vi "DVS_LabVIEW_Controller - Copy.vi"() -> ()   [LabVIEW 2013]
doc: "This example demonstrates temperature control and monitoring.\n\nNote:\nBefore start this VI is it necessary:\n\n- preconfigure some specific parameters that are not supported by this driver (e.g. PV-I/O Type, Linearization type, Alarm Input Values... ) by Quick Codes, or by Eurotherm iTools or by instrument front panel controls\n- enter correct VISA Resource Descriptor, Device Address and Baud Rate into front-panel controls"
uses:
  <vilib>/Instr/_visa.llb/VISA Event Mechanism.ctl
  <vilib>/Instr/_visa.llb/Select Event Type.ctl
  <vilib>/DAQmx/read.llb/DAQmx Read (Analog DBL 1Chan 1Samp).vi
  <vilib>/Utility/file.llb/Write To Spreadsheet File (string).vi
  <vilib>/Instr/_visa.llb/VISA Configure Serial Port (Instr).vi
  <vilib>/DAQmx/miscellaneous.llb/DAQmx Fill In Error Info.vi
  <instrlib>/Keithley 24XX/Public/Data/Read (Single Point).vi
  <instrlib>/Keithley 24XX/Keithley 24XX.lvlib
panel:
  in  "stop":bool
  in  "Tab Control":T1(tab)
  in  "Add comments to the data file here and click anywhere outside\nthe comment box to save. The time at which the comment is\nsaved is recorded in the data file.":string
  in  "O2 PUMP":bool
  in  "QCM":bool
  out "Program Errors":errorcluster
  out "Starting Date/Time":string
  in  "Keithley 4200":bool
  in  "Keithley 2420":bool
  in  "J-KEM":bool
  in  "Automatically stop\nmeasurement?":bool
  in  "Stop after elapsed minutes":dbl
  out "Time Elapsed (min)":dbl caption="Elapsed Time (s)"
  in  "RapidOX":bool
  out "Freq and Resistance Graph 2":T2(graph)
  out "Frequency (Hz)":dbl format="%.6e"
  out "Resistance (Ohm)":dbl format="%.6e"
  out "Waveform Chart 5":cluster{dbl, dbl}(graph)
  out "Current Temp (C)":dbl
  in  "Temp Setpoint (C)":dbl=25.0
  out "Current Setpoint (C)":dbl
  out "Waveform Chart 2":dbl(graph)
  out "Waveform Chart":cluster{dbl}(graph)
  out "Torr":dbl
  out "%":dbl
  out "atm":dbl
  out "O2 pump voltage":dbl format="%0.2f"
  in  "Com Port":i32(ring) items=["Com 1", "Com 2", "Com 3", "Com 4", "Com 5", "Com 6", "COM 7", "COM 8", "COM 9", "COM 10", "COM 11", "COM 12", "com 13", "COM 14"]
  in  "Baud Rate 2":i32(ring)=2 items=["2400", "4800", "9600", "19200", "38400", "57600", "115200"]
  in  "Com Port 2":i32(ring) items=["Com 1", "Com 2", "Com 3", "Com 4", "Com 5", "Com 6", "COM 7", "COM 8", "COM 9", "COM 10", "COM 11", "COM 12", "com 13", "COM 14"]
  out "Waveform Chart 6":cluster{dbl}(graph)
  out "O2 Concentration (%)":dbl
  out "Waveform Chart 4":cluster{"Resistance":sgl}(graph)
  out "Resistance (Ohm)":sgl
  in  "Measurement":enum16{"Resistor/Diode", "Transistor"}(ring)
  out "Waveform Chart 3":cluster{dbl}(graph)
  out "XY Graph":cluster{dbl[], dbl[]}(graph)
  out "Current (A)    Voltage (V)":dbl[][](array[numeric]) caption="appended array"
  out "Resistance (Ohm)":dbl
  # "Configuring Instrument\n \nPlease Wait......\n\nChart will update in 20 sec"
  # "Instruments Connected"
  # "COMMENT BOX"
  # "Instructions:\nSelect the instruments above which are connected, turned on, and configured to record data.\nRun the Pirani Control software, and make sure Pirani is saving a log of the temp/pressure/gas flow data. \nClick the RUN arrow on the LabVIEW toolbar, and wait for instruments to begin recording.\nTo end, click the red STOP button ONLY for instruments that are running.\nDO NOT press the STOP button on the toolbar."
  # "O2 Partial\nPressure"
  # "V"
  # "4-Point Resistance Measurement:\nSMU1 = Current Source, Voltmeter\nSMU2 = COM & GND"
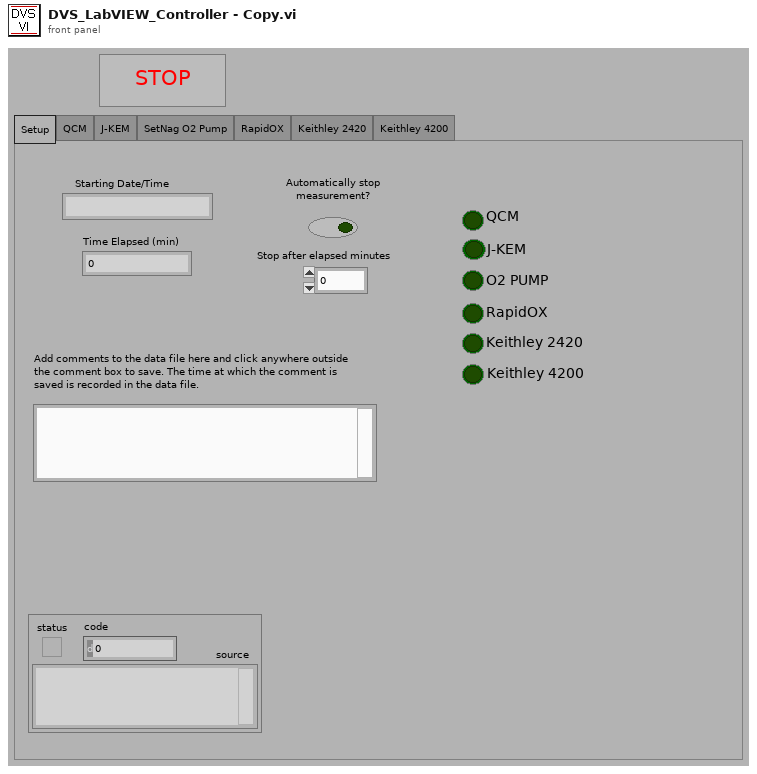
[diagram p1: front panel]
types:
  T1 = enum32{"Setup", "QCM", "J-KEM", "SetNag O2 Pump", "RapidOX", "Keithley 2420", "Keithley 4200"}
  T2 = cluster{"XY chart data":cluster{"x":dbl, "y":dbl}[]}[]
  T3 = enum16{"open", "open or create", "create or replace", "create", "open (read only)"}
  T4 = enum16{"no parity", "odd parity", "even parity", "mark parity", "space parity"}
  T5 = typedef "Select Event Type.ctl" = u32
  T6 = typedef "VISA Event Mechanism.ctl" = u16
  T7 = cluster{bool, "VISA resource name":refnum<visa-resource-name>, "error out":errorcluster}
  T8 = cluster{bool, "VISA resource name out":refnum<visa-resource-name>, "error out":errorcluster}
  T9 = cluster{"task out":refnum<k21>, "error out":errorcluster, bool}
  T10 = cluster{bool, "VISA out":refnum<visa-resource-name>, "error out":errorcluster}
  T11 = cluster{"timestamp out":dbl, "Frequency out":dbl}
  T12 = cluster{"timestamp out":dbl, "Resistance out":dbl}
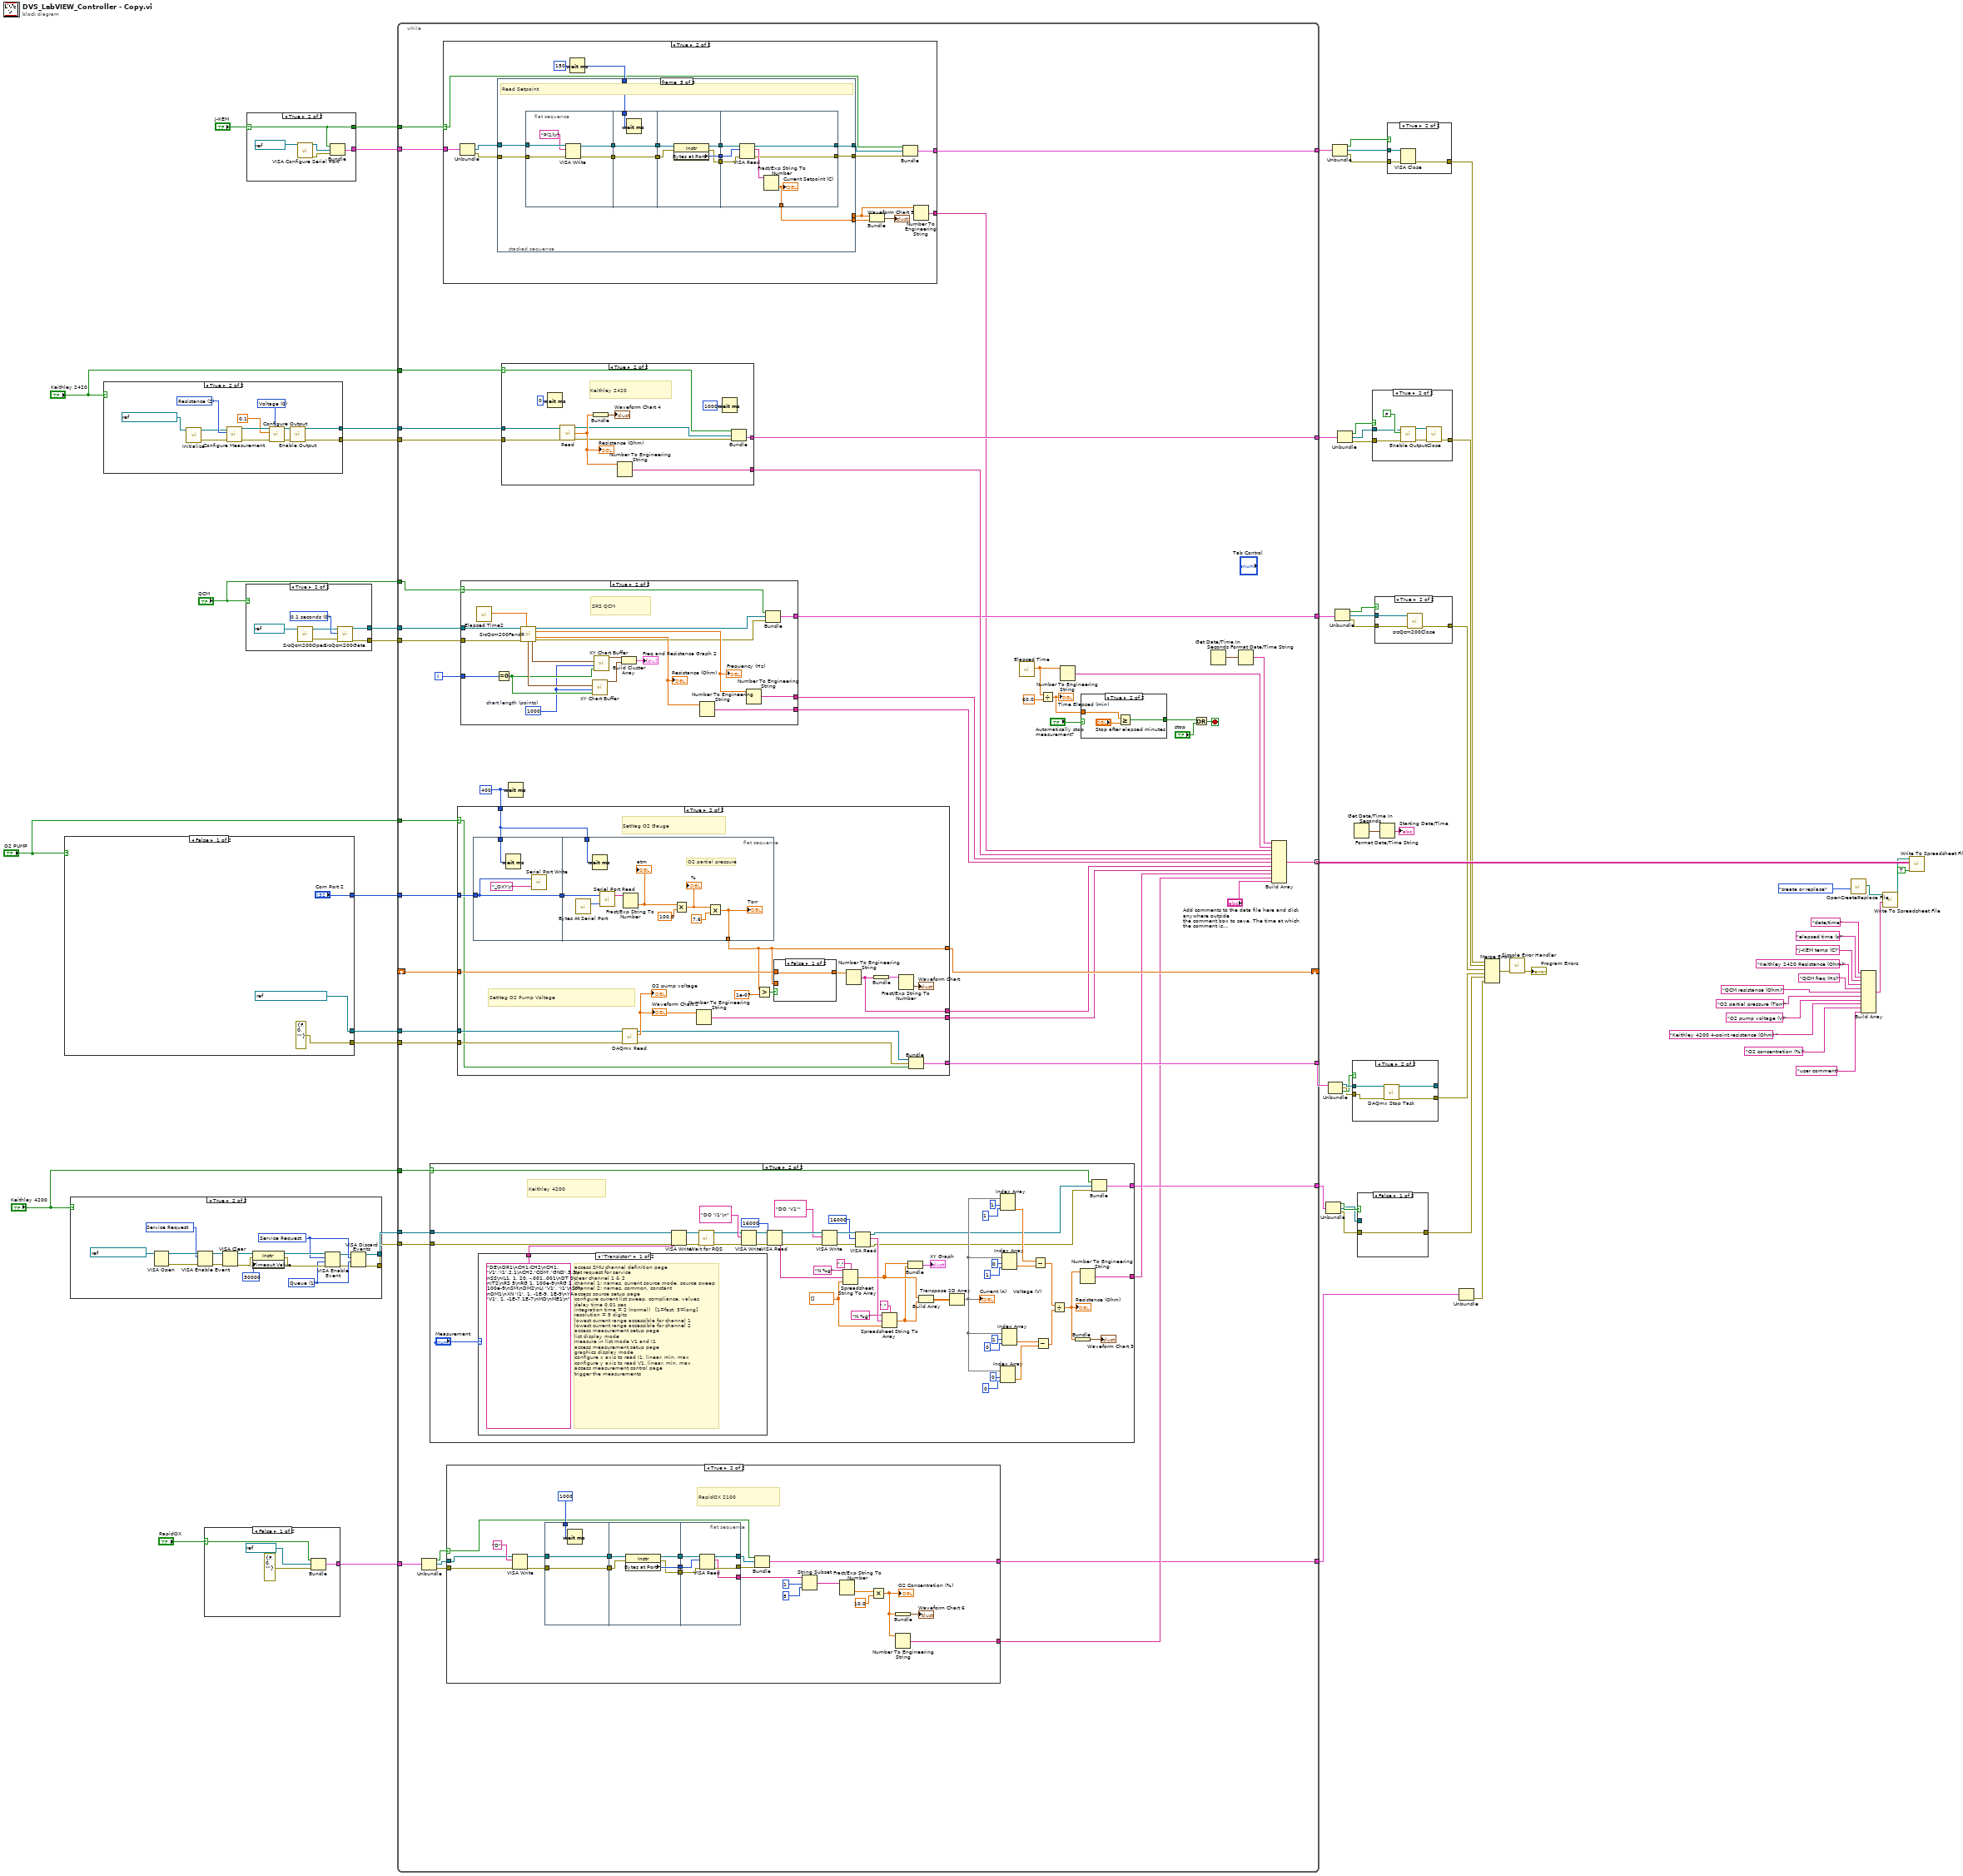
[diagram p0: block diagram]
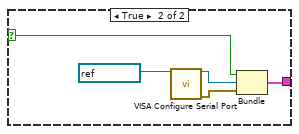
[diagram p2: hidden frame]
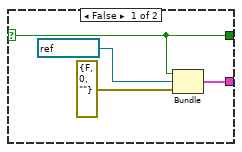
[diagram p4: hidden frame]
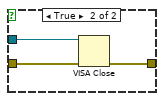
[diagram p5: hidden frame]
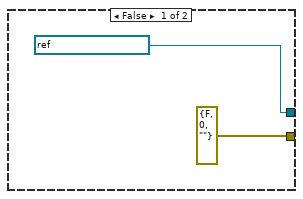
[diagram p7: hidden frame]
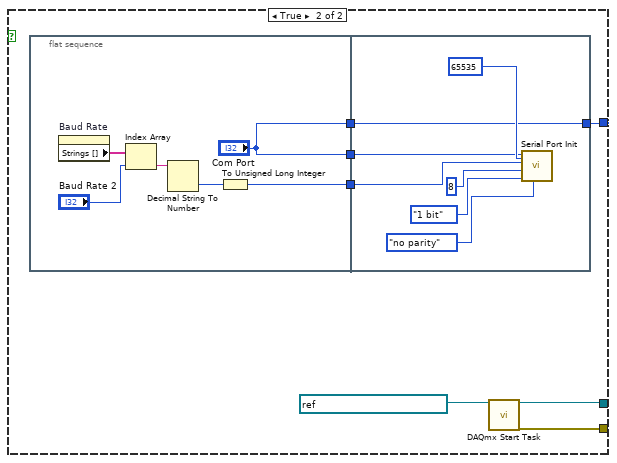
[diagram p8: hidden frame]
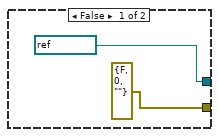
[diagram p10: hidden frame]
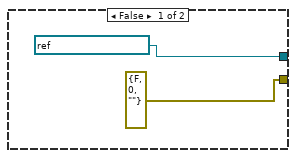
[diagram p12: hidden frame]
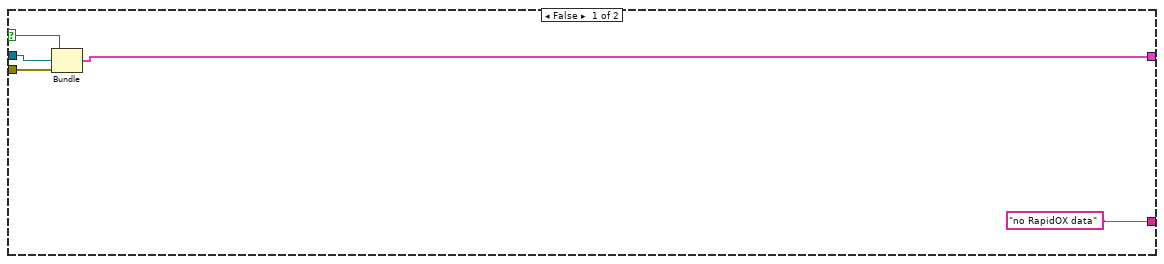
[diagram p13: hidden frame]
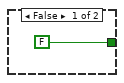
[diagram p14: hidden frame]
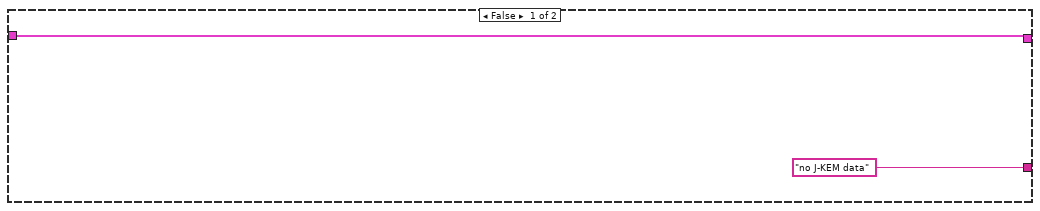
[diagram p15: hidden frame]
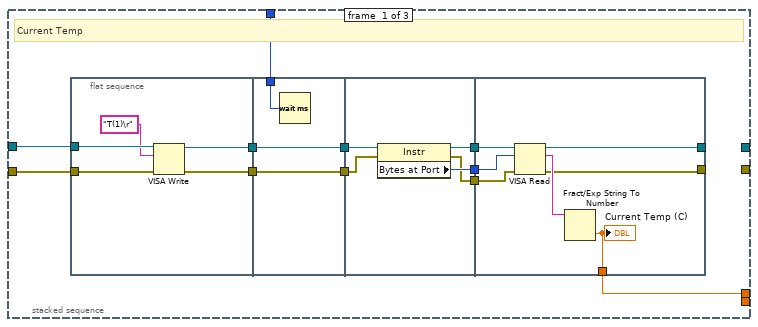
[diagram p16: hidden frame]
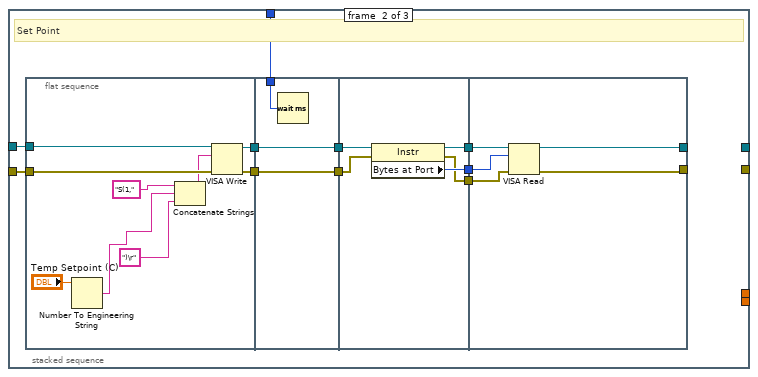
[diagram p17: hidden frame]
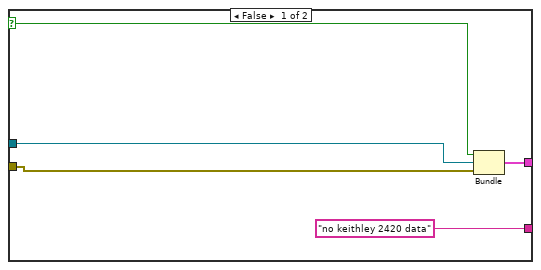
[diagram p18: hidden frame]
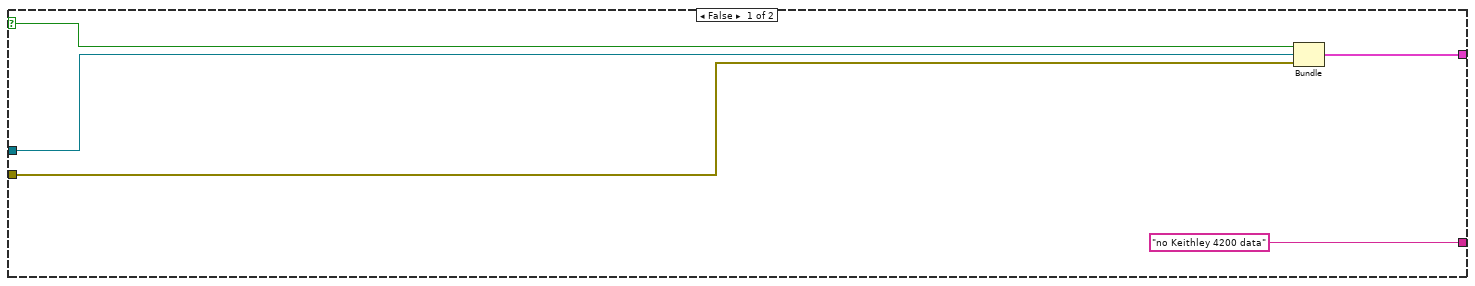
[diagram p19: hidden frame]
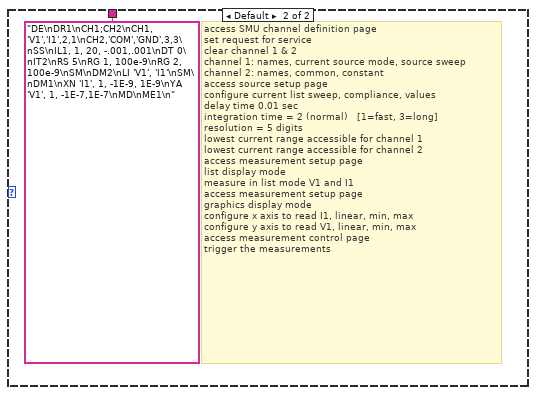
[diagram p20: hidden frame]
diagram:
  n1 = case shown="False" "O2 PUMP" {
    tunnel: ["Com Port 2" w73] -> w54
    tunnel: [refnum<k21> "SetNag_Pump_Voltage" ("task/channels in") w71] -> w53
    tunnel: [errorcluster {"status"=FALSE, "code"=0, "source"=""} ("error out") w70] -> w52
    frame False {
    }
    frame True {
      n2 = flat-sequence {
        tunnel: ["Com Port"] -> w76
        tunnel: [w78] -> w75
        tunnel: ["Com Port"] -> w74
        tunnel: w76 -> [w84]
        tunnel: w75 -> [w83]
        tunnel: w74 -> [w85]
        tunnel: [w85] -> w73
        frame #0 {
          n3 = property on="Baud Rate" class="Ring (strict)"() -> ("Strings []"=w80:string[])  [unwired: 2 in, 2 out]
          n4 = Index Array(array=w80, index="Baud Rate 2") -> (element=w81:string)
          n5 = Decimal String To Number(string=w81) -> (number=w79:i32)  [unwired: 2 in, 1 out]
          n6 = To Unsigned Long Integer(number=w79) -> (unsigned 32bit integer=w78:u32)
        }
        frame #1 {
          n7 = call <vilib>:"Serial Port Init.vi"("parity"=T4."no parity", "buffer size"=u16 65535, "stop bits"=enum16{"1 bit", "1.5 bits", "2 bits"}."1 bit", "data bits"=u16 8, "baud rate"=w83, "port number"=w84) -> ()  [unwired: 1 in, 1 out]
        }
      }
      n8 = call <vilib>:"DAQmx Start Task.vi"("task/channels in"=refnum<k21> "SetNag_Pump_Voltage") -> ("task out"=w71:refnum<k21>, "error out"=w70:errorcluster)  [unwired: 13 in]
    }
  }
  n9 = case shown="True" "Keithley 4200" {
    tunnel: [refnum<visa-resource-name> "GPIB0::17::INSTR" ("VISA resource name") w93] -> w48
    tunnel: [errorcluster {"status"=FALSE, "code"=0, "source"=""} ("error out") w92] -> w47
    frame False {
    }
    frame True {
      w105 = T5 1073684491 items=["Service Request"=1073684491, "Trigger"=3221168138, "Clear"=1073684493, "VXI Signal"=1073684512, "VXI/VME Interrupt"=3221168161, "VXI/VME Sysfail"=1073684509, "VXI/VME Sysreset"=1073684510, "GPIB CIC"=1073684498, "GPIB Talk"=1073684499, "GPIB Listen"=1073684500, "PXI Interrupt"=1073684514, "Serial Break"=1073684515, "Serial TermChar"=1073684516, "Serial CTS"=1073684521, "Serial DSR"=1073684522, "Serial DCD"=1073684524, "Serial RI"=1073684526, "Serial Character"=1073684533, "USB Interrupt"=1073684535, "All Enabled"=1073709055] ("Event Type")
      w98 = T6 1 items=["Queue"=1] ("Mechanism Type")
      w97 = T5 1073684491 items=["Service Request"=1073684491, "Trigger"=3221168138, "Clear"=1073684493, "VXI Signal"=1073684512, "VXI/VME Interrupt"=3221168161, "VXI/VME Sysfail"=1073684509, "VXI/VME Sysreset"=1073684510, "GPIB CIC"=1073684498, "GPIB Talk"=1073684499, "GPIB Listen"=1073684500, "PXI Interrupt"=1073684514, "Serial Break"=1073684515, "Serial TermChar"=1073684516, "Serial CTS"=1073684521, "Serial DSR"=1073684522, "Serial DCD"=1073684524, "Serial RI"=1073684526, "Serial Character"=1073684533, "USB Interrupt"=1073684535, "All Enabled"=1073709055] ("Event Type")
      n10 = VISA Open(VISA resource name=refnum<visa-resource-name> "GPIB0::17::INSTR") -> (VISA resource name=w107:refnum<visa-resource-name>, error out=w108:errorcluster)  [unwired: 1 in, 3 out]
      n11 = VISA Enable Event(8:w108, 10:w105, 11:w107) -> (0:w104:errorcluster, 3:w103:refnum<visa-resource-name>)  [unwired: 1 out]
      n12 = VISA Clear(VISA resource name=w103, error in (no error)=w104) -> (VISA resource name out=w99:refnum<visa-resource-name>, error out=w100:errorcluster)
      n13 = property class="Instr"(reference=w99, error in=w100, "General Settings:Timeout Value"=u32 30000) -> (reference out=w101:refnum<visa-resource-name>, error out=w102:errorcluster)
      n14 = VISA Enable Event(8:w102, 9:w98, 10:w97, 11:w101) -> (0:w96:errorcluster, 3:w95:refnum<visa-resource-name>)
      n15 = VISA Discard Events(8:w96, 9:w98, 10:w97, 11:w95) -> (0:w92:errorcluster, 3:w93:refnum<visa-resource-name>)
    }
  }
  n16 = case shown="True" "Keithley 2420" {
    tunnel: [refnum<visa-resource-name> "GPIB1::24::INSTR" ("VISA resource name") w112] -> w60
    tunnel: [errorcluster {"status"=FALSE, "code"=0, "source"=""} ("error out") w111] -> w59
    frame False {
    }
    frame True {
      w116 = u16 0 items=["Voltage", "Current"] ("Source Mode  (0: Voltage)")
      w121 = u16 2 items=["Volts", "Current", "Resistance"] ("Function (0: Volts)")
      n17 = call <instrlib>:"Initialize.vi"("VISA resource name"=refnum<visa-resource-name> "GPIB1::24::INSTR") -> ("error out"=w113:errorcluster, "VISA resource name out"=w114:refnum<visa-resource-name>)  [unwired: 9 in]
      n18 = call <instrlib>:"Configure Measurement.vi"("error in (no error)"=w113, "Function (0: Volts)"=w121, "VISA resource name"=w114) -> ("error out"=w120:errorcluster, "VISA resource name out"=w119:refnum<visa-resource-name>)  [unwired: 7 in]
      n19 = call <instrlib>:"Configure Output.vi"("Source Mode  (0: Voltage)"=w116, "error in (no error)"=w120, "Output Level (0)"=0.1, "VISA resource name"=w119) -> ("error out"=w118:errorcluster, "VISA resource name out"=w117:refnum<visa-resource-name>)  [unwired: 6 in]
      n20 = call <instrlib>:"Enable Output.vi"("error in (no error)"=w118, "VISA resource name"=w117) -> ("error out"=w111:errorcluster, "VISA resource name out"=w112:refnum<visa-resource-name>)  [unwired: 8 in]
    }
  }
  n21 = case shown="False" "RapidOX" {
    selector: "RapidOX" -> [w123 w127]
    tunnel: [w124 w128] -> w4
    frame False {
      n22 = Bundle(w123, "VISA resource name"=refnum<visa-resource-name> "COM7", "error out"=errorcluster {"status"=FALSE, "code"=0, "source"=""}) -> (w124:T7)  [unwired: 1 in]
    }
    frame True {
      n23 = call-poly "VISA Configure Serial Port"("VISA resource name"=refnum<visa-resource-name> "COM7") -> ("VISA resource name out"=w130:refnum<visa-resource-name>, "error out"=w129:errorcluster)  [unwired: 13 in]
      n24 = Bundle(w127, "VISA resource name out"=w130, "error out"=w129) -> (w128:T8)  [unwired: 1 in]
    }
  }
  n25 = case shown="True" "QCM" {
    tunnel: [refnum<visa-resource-name> "COM6" ("VISA in") w135] -> w58
    tunnel: [errorcluster {"status"=FALSE, "code"=0, "source"=""} ("error out") w134] -> w57
    frame False {
    }
    frame True {
      w139 = u16 0 items=["0.1 seconds", "1.0 seconds", "10.0 seconds"] ("Gate in")
      n26 = call <instrlib>:"SrsQcm200Open.vi"("VISA in"=refnum<visa-resource-name> "COM6") -> ("error out"=w136:errorcluster, "VISA out"=w137:refnum<visa-resource-name>)  [unwired: 4 in]
      n27 = call <instrlib>:"SrsQcm200Gate.vi"("VISA in"=w137, "Gate in"=w139, "error in (no error)"=w136) -> ("VISA out"=w135:refnum<visa-resource-name>, "error out"=w134:errorcluster)  [unwired: 14 in, 1 out]
    }
  }
  n28 = case shown="True" "J-KEM" {
    selector: "J-KEM" -> [w140 w144]
    tunnel: [w141 w145] -> w29
    tunnel: [w140 w144] -> w21
    frame False {
      n29 = Bundle(w140, "VISA resource name"=refnum<visa-resource-name> "COM3", "error out"=errorcluster {"status"=FALSE, "code"=0, "source"=""}) -> (w141:T7)  [unwired: 1 in]
    }
    frame True {
      n30 = call-poly "VISA Configure Serial Port"("VISA resource name"=refnum<visa-resource-name> "COM3") -> ("VISA resource name out"=w147:refnum<visa-resource-name>, "error out"=w146:errorcluster)  [unwired: 13 in]
      n31 = Bundle(w144, "VISA resource name out"=w147, "error out"=w146) -> (w145:T8)  [unwired: 1 in]
    }
  }
  n32 = while {
    shift-right: [w195] -> _
    shift-left: _ -> [w194]
    tunnel: [w190] -> w62 mode=indexing
    tunnel: "Keithley 2420" -> [w186]
    tunnel: w60 -> [w188]
    tunnel: w59 -> [w187]
    tunnel: w58 -> [w185]
    tunnel: w57 -> [w184]
    tunnel: "QCM" -> [w182]
    tunnel: "O2 PUMP" -> [w168]
    tunnel: w54 -> [w181]
    tunnel: w53 -> [w180]
    tunnel: w52 -> [w179]
    tunnel: "Keithley 4200" -> [w172]
    tunnel: w48 -> [w178]
    tunnel: w47 -> [w177]
    tunnel: [w170] -> w45
    tunnel: [w169] -> w41
    tunnel: [w167] -> w37
    tunnel: [w166] -> w33
    tunnel: w29 -> [w165]
    tunnel: [w164] -> w27
    tunnel: w21 -> [w162]
    tunnel: w4 -> [w154]
    tunnel: [w149] -> w2
    i -> [w193]
    stop <- w160 stop-if-true
    w192 = u32 400 ("milliseconds to wait")
    n33 = Unbundle(w154) -> (w153:bool, "VISA resource name out"=w152:refnum<visa-resource-name>, "error out"=w151:errorcluster)
    n34 = case shown="True" w172 {
      selector: w172 -> [w372 w378]
      tunnel: w178 -> [w374 w383]
      tunnel: w177 -> [w373 w382]
      tunnel: ["no Keithley 4200 data" w381] -> w173
      tunnel: [w371 w377] -> w166
      frame False {
        n35 = Bundle(w372, "VISA resource name"=w374, "error out"=w373) -> (w371:T7)  [unwired: 1 in]
      }
      frame True {
        w416 = dbl[] []
        # "Keithley 4200"
        n36 = case shown="\"Transistor\"" "Measurement" {
          tunnel: ["DE\nDR1\nCH1;CH2\nCH1, 'V1','I1',2,1\nCH2,'COM','GND',3,3\nSS\nIL1, 1, 20, -.001,.001\nDT 0\nIT2\nRS 5\nRG 1, 100e-9\nRG 2, 100e-9\nSM\nDM2\nLI 'V1', 'I1'\nSM\nDM1\nXN 'I1', 1, -1E-9, 1E-9\nYA 'V1', 1, -1E-7,1E-7\nMD\nME1\n" ("write buffer") "DE\nDR1\nCH1;CH2\nCH1, 'V1','I1',2,1\nCH2,'COM','GND',3,3\nSS\nIL1, 1, 20, -.001,.001\nDT 0\nIT2\nRS 5\nRG 1, 100e-9\nRG 2, 100e-9\nSM\nDM2\nLI 'V1', 'I1'\nSM\nDM1\nXN 'I1', 1, -1E-9, 1E-9\nYA 'V1', 1, -1E-7,1E-7\nMD\nME1\n" ("write buffer")] -> w390
          frame "Transistor" {
            # "access SMU channel definition page\nset request for service\nclear channel 1 & 2\nchannel 1: names, current source mode, source sweep\nchannel 2: names, common, constant\naccess source setup page\nconfigure current list sweep, compliance, values\ndelay time 0.01 sec\nintegration time = 2 (normal)   [1=fast, 3=long]\nresolution = 5 digits\nlowest current range accessible for channel 1\nlowest current range accessible for channel 2\naccess measurement setup page\nlist display mode\nmeasure in list mode V1 and I1\naccess measurement setup page\ngraphics display mode\nconfigure x axis to read I1, linear, min, max\nconfigure y axis to read V1, linear, min, max\naccess measurement control page\ntrigger the measurements"
          }
          frame Default {
            # "access SMU channel definition page\nset request for service\nclear channel 1 & 2\nchannel 1: names, current source mode, source sweep\nchannel 2: names, common, constant\naccess source setup page\nconfigure current list sweep, compliance, values\ndelay time 0.01 sec\nintegration time = 2 (normal)   [1=fast, 3=long]\nresolution = 5 digits\nlowest current range accessible for channel 1\nlowest current range accessible for channel 2\naccess measurement setup page\nlist display mode\nmeasure in list mode V1 and I1\naccess measurement setup page\ngraphics display mode\nconfigure x axis to read I1, linear, min, max\nconfigure y axis to read V1, linear, min, max\naccess measurement control page\ntrigger the measurements"
          }
        }
        n37 = VISA Write(VISA resource name=w383, write buffer=w390, error in (no error)=w382) -> (VISA resource name out=w391:refnum<visa-resource-name>, error out=w392:errorcluster)  [unwired: 1 out]
        n38 = call <vilib>:"Wait for RQS.vi"("error in (no error)"=w392, "VISA resource name"=w391) -> ("error out"=w388:errorcluster, "VISA resource name out"=w389:refnum<visa-resource-name>)  [unwired: 1 in, 7 out]
        n39 = VISA Write(VISA resource name=w389, write buffer="DO 'I1'\n", error in (no error)=w388) -> (VISA resource name out=w426:refnum<visa-resource-name>, error out=w422:errorcluster)  [unwired: 1 out]
        n40 = VISA Read(VISA resource name=w426, byte count=u32 16000, error in (no error)=w422) -> (VISA resource name out=w424:refnum<visa-resource-name>, read buffer=w409:string, error out=w420:errorcluster)  [unwired: 1 out]
        n41 = VISA Write(VISA resource name=w424, write buffer="DO 'V1'", error in (no error)=w420) -> (VISA resource name out=w418:refnum<visa-resource-name>, error out=w419:errorcluster)  [unwired: 1 out]
        n42 = Spreadsheet String To Array(delimiter (Tab)=",", format string="N %g", spreadsheet string=w409, array type (2D Dbl)=w416) -> (array=w413:dbl[])
        n43 = VISA Read(VISA resource name=w418, byte count=u32 16000, error in (no error)=w419) -> (VISA resource name out=w380:refnum<visa-resource-name>, read buffer=w408:string, error out=w379:errorcluster)  [unwired: 1 out]
        n44 = Spreadsheet String To Array(delimiter (Tab)=",", format string="N %g", spreadsheet string=w408, array type (2D Dbl)=w416) -> (array=w412:dbl[])
        n45 = Bundle(w413, w412) -> (→"XY Graph":cluster{dbl[], dbl[]})  [unwired: 1 in]
        n46 = Build Array(w413, w412) -> (w410:dbl[][])
        n47 = Transpose 2D Array(2D array=w410) -> (transposed array=w395:dbl[][])
        "Current (A)    Voltage (V)" <- w395
        n48 = Index Array(array=w395, index (row)=1, index (col)=1 ("index (row)")) -> (element=w397:dbl)
        n49 = Index Array(array=w395, index (row)=0, index (col)=0 ("index (row)")) -> (element=w398:dbl)
        n50 = Index Array(array=w395, index (row)=0, index (col)=1 ("index (row)")) -> (element=w396:dbl)
        n51 = Index Array(array=w395, index (row)=1, index (col)=0 ("index (row)")) -> (element=w399:dbl)
        n52 = Subtract(x=w397, y=w396) -> (x-y=w393:dbl)
        n53 = Subtract(x=w399, y=w398) -> (x-y=w394:dbl)
        n54 = Divide(x=w393, y=w394) -> (x/y=w384:dbl)
        "Resistance (Ohm)" <- w384
        n55 = Bundle(w384) -> (→"Waveform Chart 3":cluster{dbl})  [unwired: 1 in]
        n56 = Number To Engineering String(4:w384) -> (0:w381:string)  [unwired: 3 in]
        n57 = Bundle(w378, "VISA resource name out"=w380, "error out"=w379) -> (w377:T8)  [unwired: 1 in]
      }
    }
    n58 = case shown="True" w162 {
      selector: w162 -> [_ w247]
      tunnel: w165 -> [w246 w253]
      tunnel: [w246 w250] -> w164
      tunnel: ["no J-KEM data" w248] -> w163
      frame False {
      }
      frame True {
        w258 = u32 150 ("milliseconds to wait")
        n59 = Unbundle(w253) -> ("VISA resource name out"=w252:refnum<visa-resource-name>, "error out"=w251:errorcluster)  [unwired: 1 out]
        n60 = stacked-sequence {
          tunnel: w252 -> [w262 w292 w326]
          tunnel: w251 -> [w261 w291 w325]
          tunnel: w258 -> [w260 w290 w327]
          tunnel: [_ _ w324] -> w254
          tunnel: [_ _ w323] -> w255
          tunnel: [w259 _ _] -> w249
          tunnel: [_ _ w322] -> w257
          frame #0 {
            # "Current Temp"
            n61 = flat-sequence {
              tunnel: w262 -> [w274]
              tunnel: w261 -> [w273]
              tunnel: [w271] -> w269
              tunnel: [w270] -> w268
              tunnel: w260 -> [w277]
              tunnel: [w276] -> w267
              tunnel: w269 -> [w276]
              tunnel: w268 -> [w275]
              tunnel: [w275] -> w266
              tunnel: w267 -> [w282]
              tunnel: w266 -> [w281]
              tunnel: [w280] -> w265
              tunnel: [w279] -> w264
              tunnel: [w278] -> w263
              tunnel: w265 -> [w289]
              tunnel: w264 -> [w288]
              tunnel: w263 -> [w287]
              tunnel: [w284] -> _
              tunnel: [w285] -> _
              tunnel: [w283] -> w259
              frame #0 {
                n62 = VISA Write(VISA resource name=w274, write buffer="T(1)\r", error in (no error)=w273) -> (VISA resource name out=w271:refnum<visa-resource-name>, error out=w270:errorcluster)  [unwired: 1 out]
              }
              frame #1 {
                n63 = Wait (ms)(milliseconds to wait=w277) -> ()  [unwired: 1 out]
              }
              frame #2 {
                n64 = property class="Instr"(reference=w282, error in=w281) -> (reference out=w280:refnum<visa-resource-name>, error out=w278:errorcluster, "Bytes at Port"=w279:u32)
              }
              frame #3 {
                n65 = VISA Read(VISA resource name=w289, byte count=w288, error in (no error)=w287) -> (VISA resource name out=w285:refnum<visa-resource-name>, read buffer=w286:string, error out=w284:errorcluster)  [unwired: 1 out]
                n66 = Fract/Exp String To Number(string=w286) -> (number=w283:dbl)  [unwired: 3 in, 1 out]
                "Current Temp (C)" <- w283
              }
            }
          }
          frame #1 {
            # "Set Point"
            n67 = flat-sequence {
              tunnel: w292 -> [w308]
              tunnel: w291 -> [w307]
              tunnel: [w306] -> w299
              tunnel: [w305] -> w298
              tunnel: w290 -> [w311]
              tunnel: [w310] -> w297
              tunnel: w299 -> [w310]
              tunnel: w298 -> [w309]
              tunnel: [w309] -> w296
              tunnel: w297 -> [w316]
              tunnel: w296 -> [w315]
              tunnel: [w314] -> w295
              tunnel: [w313] -> w294
              tunnel: [w312] -> w293
              tunnel: w295 -> [w321]
              tunnel: w294 -> [w320]
              tunnel: w293 -> [w319]
              tunnel: [w317] -> _
              tunnel: [w318] -> _
              frame #0 {
                n68 = Number To Engineering String(4:"Temp Setpoint (C)") -> (0:w301:string)  [unwired: 3 in]
                n69 = Concatenate Strings("S(1," ("write buffer"), w301, ")\r" ("write buffer")) -> (w304:string)
                n70 = VISA Write(VISA resource name=w308, write buffer=w304, error in (no error)=w307) -> (VISA resource name out=w306:refnum<visa-resource-name>, error out=w305:errorcluster)  [unwired: 1 out]
              }
              frame #1 {
                n71 = Wait (ms)(milliseconds to wait=w311) -> ()  [unwired: 1 out]
              }
              frame #2 {
                n72 = property class="Instr"(reference=w316, error in=w315) -> (reference out=w314:refnum<visa-resource-name>, error out=w312:errorcluster, "Bytes at Port"=w313:u32)
              }
              frame #3 {
                n73 = VISA Read(VISA resource name=w321, byte count=w320, error in (no error)=w319) -> (VISA resource name out=w318:refnum<visa-resource-name>, error out=w317:errorcluster)  [unwired: 2 out]
              }
            }
          }
          frame #2 {
            # "Read Setpoint"
            n74 = flat-sequence {
              tunnel: w326 -> [w339]
              tunnel: w325 -> [w338]
              tunnel: [w336] -> w334
              tunnel: [w335] -> w333
              tunnel: [w342] -> w332
              tunnel: w334 -> [w342]
              tunnel: w333 -> [w341]
              tunnel: [w341] -> w331
              tunnel: w327 -> [w340]
              tunnel: w332 -> [w347]
              tunnel: w331 -> [w346]
              tunnel: [w345] -> w330
              tunnel: [w344] -> w329
              tunnel: [w343] -> w328
              tunnel: w330 -> [w354]
              tunnel: w329 -> [w353]
              tunnel: w328 -> [w352]
              tunnel: [w349] -> w323
              tunnel: [w350] -> w324
              tunnel: [w348] -> w322
              frame #0 {
                n75 = VISA Write(VISA resource name=w339, write buffer="P(1)\r", error in (no error)=w338) -> (VISA resource name out=w336:refnum<visa-resource-name>, error out=w335:errorcluster)  [unwired: 1 out]
              }
              frame #1 {
                n76 = Wait (ms)(milliseconds to wait=w340) -> ()  [unwired: 1 out]
              }
              frame #2 {
                n77 = property class="Instr"(reference=w347, error in=w346) -> (reference out=w345:refnum<visa-resource-name>, error out=w343:errorcluster, "Bytes at Port"=w344:u32)
              }
              frame #3 {
                n78 = VISA Read(VISA resource name=w354, byte count=w353, error in (no error)=w352) -> (VISA resource name out=w350:refnum<visa-resource-name>, read buffer=w351:string, error out=w349:errorcluster)  [unwired: 1 out]
                n79 = Fract/Exp String To Number(string=w351) -> (number=w348:dbl)  [unwired: 3 in, 1 out]
                "Current Setpoint (C)" <- w348
              }
            }
          }
        }
        n80 = Wait (ms)(milliseconds to wait=w258) -> ()  [unwired: 1 out]
        n81 = Bundle(w249, w257) -> (→"Waveform Chart 5":cluster{dbl, dbl})  [unwired: 1 in]
        n82 = Bundle(w247, "VISA resource name out"=w254, "error out"=w255) -> (w250:T8)  [unwired: 1 in]
        n83 = Number To Engineering String(4:w249) -> (0:w248:string)  [unwired: 3 in]
      }
    }
    n84 = case shown="True" w153 {
      selector: w153 -> [w200 w207]
      tunnel: w152 -> [w201 w206]
      tunnel: w151 -> [w199 w205]
      tunnel: ["no RapidOX data" w204] -> w150
      tunnel: [w198 w203] -> w149
      frame False {
        n85 = Bundle(w200, "VISA resource name out"=w201, "error out"=w199) -> (w198:T8)  [unwired: 1 in]
      }
      frame True {
        # "RapidOX 2100"
        n86 = VISA Write(VISA resource name=w206, write buffer="D", error in (no error)=w205) -> (VISA resource name out=w217:refnum<visa-resource-name>, error out=w216:errorcluster)  [unwired: 1 out]
        n87 = flat-sequence {
          tunnel: [w228] -> w226
          tunnel: [w227] -> w225
          tunnel: u32 1000 ("milliseconds to wait") -> [w229]
          tunnel: w217 -> [w228]
          tunnel: w216 -> [w227]
          tunnel: w226 -> [w234]
          tunnel: w225 -> [w233]
          tunnel: [w232] -> w224
          tunnel: [w231] -> w223
          tunnel: [w230] -> w222
          tunnel: w224 -> [w240]
          tunnel: w223 -> [w239]
          tunnel: w222 -> [w238]
          tunnel: [w236] -> w220
          tunnel: [w237] -> w221
          tunnel: [w235] -> w208
          frame #0 {
            n88 = Wait (ms)(milliseconds to wait=w229) -> ()  [unwired: 1 out]
          }
          frame #1 {
            n89 = property class="Instr"(reference=w234, error in=w233) -> (reference out=w232:refnum<visa-resource-name>, error out=w230:errorcluster, "Bytes at Port"=w231:u32)
          }
          frame #2 {
            n90 = VISA Read(VISA resource name=w240, byte count=w239, error in (no error)=w238) -> (VISA resource name out=w237:refnum<visa-resource-name>, read buffer=w235:string, error out=w236:errorcluster)  [unwired: 1 out]
          }
        }
        n91 = Bundle(w207, "VISA resource name out"=w221, "error out"=w220) -> (w203:T8)  [unwired: 1 in]
        n92 = String Subset(string=w208, offset (0)=1, length (rest)=5 ("length (rest)")) -> (substring=w211:string)
        n93 = Fract/Exp String To Number(string=w211) -> (number=w213:dbl)  [unwired: 3 in, 1 out]
        n94 = Multiply(x=w213, y=10.0) -> (x*y=w215:dbl)
        "O2 Concentration (%)" <- w215
        n95 = Bundle(w215) -> (→"Waveform Chart 6":cluster{dbl})  [unwired: 1 in]
        n96 = Number To Engineering String(4:w215) -> (0:w204:string)  [unwired: 3 in]
      }
    }
    n97 = case shown="True" w168 {
      selector: w168 -> [w454 w460]
      tunnel: [w458 w468] -> w195
      tunnel: w194 -> [w458 w471]
      tunnel: w192 -> [_ w469]
      tunnel: w181 -> [_ w467]
      tunnel: w180 -> [w456 w466]
      tunnel: w179 -> [w455 w465]
      tunnel: [w457 w464] -> w176
      tunnel: [w457 w463] -> w175
      tunnel: [w453 w459] -> w167
      frame False {
        w457 = "no GenAir data"
        n98 = Bundle("task out"=w456, "error out"=w455, w454) -> (w453:T9)  [unwired: 1 in]
      }
      frame True {
        # "SetNag O2 Gauge"
        # "SetNag O2 Pump Voltage"
        n99 = flat-sequence {
          tunnel: [w480] -> w477
          tunnel: w469 -> [w482]
          tunnel: w467 -> [w480]
          tunnel: w477 -> [w483]
          tunnel: w469 -> [w490]
          tunnel: [w486] -> w468
          frame #0 {
            n100 = Wait (ms)(milliseconds to wait=w482) -> ()  [unwired: 1 out]
            n101 = call <vilib>:"Serial Port Write.vi"("string to write"="_OXY\r" ("O2 partial press"), "port number"=w480) -> ()  [unwired: 1 out]
          }
          frame #1 {
            # "O2 partial pressure"
            n102 = call <vilib>:"Bytes At Serial Port.vi"() -> ("byte count"=w491:u32)  [unwired: 1 in, 1 out]
            n103 = Wait (ms)(milliseconds to wait=w490) -> ()  [unwired: 1 out]
            n104 = call <vilib>:"Serial Port Read.vi"("requested byte count"=w491, "port number"=w483) -> ("string read"=w489:string)  [unwired: 1 out]
            n105 = Fract/Exp String To Number(string=w489) -> (number=w487:dbl)  [unwired: 3 in, 1 out]
            "atm" <- w487
            n106 = Multiply(x=w487, y=100.0) -> (x*y=w484:dbl)
            "%" <- w484
            n107 = Multiply(x=w484, y=7.6) -> (x*y=w486:dbl)
            "Torr" <- w486
          }
        }
        n108 = call-poly <vilib>:"DAQmx Read.vi"("task/channels in"=w466, "error in"=w465) -> ("task out"=w462:refnum<k21>, "data"=w470:dbl, "error out"=w461:errorcluster)  [unwired: 11 in]
        "Waveform Chart 2" <- w470
        "O2 pump voltage" <- w470
        n109 = Number To Engineering String(4:w470) -> (0:w463:string)  [unwired: 3 in]
        n110 = Greater?(x=w468, y=1e-07) -> (0:w473:bool)
        n111 = case shown="False" w473 {
          tunnel: [w478 w479] -> w472
          tunnel: w468 -> [_ w479]
          tunnel: w471 -> [w478 _]
          frame False {
          }
          frame True {
          }
        }
        n112 = Number To Engineering String(4:w472) -> (0:w464:string)  [unwired: 3 in]
        n113 = Bundle(w464) -> (w475:cluster{string})  [unwired: 1 in]
        n114 = Fract/Exp String To Number(string=w475) -> (number=→"Waveform Chart":cluster{dbl})  [unwired: 3 in, 1 out]
        n115 = Bundle("task out"=w462, "error out"=w461, w460) -> (w459:T9)  [unwired: 1 in]
      }
    }
    n116 = case shown="True" w182 {
      selector: w182 -> [w432 w435]
      tunnel: w193 -> [_ w444]
      tunnel: w185 -> [w431 w441]
      tunnel: w184 -> [w430 w440]
      tunnel: [w433 w439] -> w183
      tunnel: [w433 w438] -> w174
      tunnel: [w429 w434] -> w169
      frame False {
        w433 = "no QCM data"
        n117 = Bundle(w432, "VISA out"=w431, "error out"=w430) -> (w429:T10)  [unwired: 1 in]
      }
      frame True {
        w443 = 1000  # chart length (points)
        # "SRS QCM"
        n118 = call "Elapsed Time2"() -> ("Elapsed Time (s)"=w442:dbl)  [unwired: 12 in, 7 out]
        n119 = Equal To 0?(x=w444) -> (x = 0?=w447:bool)
        n120 = call <instrlib>:"SrsQcm200FandR.vi"("VISA in"=w441, "Reference time in"=w442, "error in (no error)"=w440) -> ("VISA out"=w437:refnum<visa-resource-name>, "Frequency out"=w446:dbl, "Resistance out"=w445:dbl, "F vs T out"=w452:T11, "R vs T out"=w451:T12, "error out"=w436:errorcluster)  [unwired: 6 in, 1 out]
        "Frequency (Hz)" <- w446
        "Resistance (Ohm)" <- w445
        n121 = call <instrlib>:"XY Chart Buffer.vi"("clear first (no:F)"=w447, "chart length (points)"=w443, "new point"=w452) -> ("XY chart data"=w449:cluster{"x":dbl, "y":dbl}[])  [unwired: 8 in]
        n122 = call <instrlib>:"XY Chart Buffer.vi"("clear first (no:F)"=w447, "chart length (points)"=w443, "new point"=w451) -> ("XY chart data"=w450:cluster{"x":dbl, "y":dbl}[])  [unwired: 8 in]
        n123 = Build Cluster Array(w450, w449) -> (→"Freq and Resistance Graph 2":T2)
        n124 = Number To Engineering String(4:w445) -> (0:w438:string)  [unwired: 3 in]
        n125 = Number To Engineering String(4:w446) -> (0:w439:string)  [unwired: 3 in]
        n126 = Bundle(w435, "VISA out"=w437, "error out"=w436) -> (w434:T10)  [unwired: 1 in]
      }
    }
    n127 = case shown="True" w186 {
      selector: w186 -> [w358 w364]
      tunnel: w188 -> [w357 w366]
      tunnel: w187 -> [w356 w367]
      tunnel: [w355 w362] -> w170
      tunnel: ["no keithley 2420 data" w361] -> w171
      frame False {
        n128 = Bundle(w358, "VISA resource name out"=w357, "error out"=w356) -> (w355:T8)  [unwired: 1 in]
      }
      frame True {
        # "Keithley 2420"
        n129 = Wait (ms)(milliseconds to wait=u32 0) -> ()  [unwired: 1 out]
        n130 = call-poly <instrlib>:"Read.vi"("VISA resource name"=w366, "error in (no error)"=w367) -> ("VISA resource name out"=w365:refnum<visa-resource-name>, "Resistance"=w369:sgl, "error out"=w363:errorcluster)  [unwired: 7 in, 4 out]
        "Resistance (Ohm)" <- w369
        n131 = Bundle("Resistance"=w369) -> (→"Waveform Chart 4":cluster{"Resistance":sgl})  [unwired: 1 in]
        n132 = Number To Engineering String(4:w369) -> (0:w361:string)  [unwired: 3 in]
        n133 = Wait (ms)(milliseconds to wait=u32 1000) -> ()  [unwired: 1 out]
        n134 = Bundle(w364, "VISA resource name out"=w365, "error out"=w363) -> (w362:T8)  [unwired: 1 in]
      }
    }
    n135 = Wait (ms)(milliseconds to wait=w192) -> ()  [unwired: 1 out]
    n136 = call "Elapsed Time"() -> ("Elapsed Time (s)"=w159:dbl)  [unwired: 12 in, 7 out]
    n137 = Divide(x=w159, y=60.0) -> (x/y=w157:dbl)
    "Time Elapsed (min)" <- w157
    n138 = Number To Engineering String(4:w159) -> (0:w196:string)  [unwired: 3 in]
    n139 = case shown="True" "Automatically stop\nmeasurement?" {
      tunnel: w157 -> [_ w243]
      tunnel: [FALSE w242] -> w155
      frame False {
      }
      frame True {
        n140 = Greater Or Equal?(x=w243, y="Stop after elapsed minutes") -> (x >= y?=w242:bool)
      }
    }
    n141 = Or(x=w155, y="stop") -> (x .or. y?=w160:bool)
    n142 = Get Date/Time In Seconds() -> (seconds since 1Jan1904=w197:timestamp)
    n143 = Format Date/Time String(seconds (now)=w197) -> (date/time string=w189:string)  [unwired: 2 in]
    n144 = Build Array(w189, w196, w163, w171, w183, w174, w176, w175, w173, w150, "Add comments to the data file here and click anywhere outside\nthe comment box to save. The time at which the comment is\nsaved is recorded in the data file.") -> (w190:string[])
  }
  n145 = Unbundle(w33) -> (w32:bool, "VISA resource name out"=w31:refnum<visa-resource-name>, "error out"=w30:errorcluster)
  n146 = Unbundle(w37) -> ("task out"=w36:refnum<k21>, "error out"=w34:errorcluster, w35:bool)
  n147 = Unbundle(w27) -> (w26:bool, "VISA resource name out"=w25:refnum<visa-resource-name>, "error out"=w24:errorcluster)
  n148 = Unbundle(w41) -> (w40:bool, "VISA out"=w39:refnum<visa-resource-name>, "error out"=w38:errorcluster)
  n149 = Unbundle(w45) -> (w44:bool, "VISA resource name out"=w43:refnum<visa-resource-name>, "error out"=w42:errorcluster)
  n150 = case shown="True" w35 {
    tunnel: [w493 w497] -> _
    tunnel: [w492 w496] -> w46
    tunnel: w36 -> [w493 w495]
    tunnel: w34 -> [w492 w494]
    frame False {
    }
    frame True {
      n151 = call <vilib>:"DAQmx Stop Task.vi"("task/channels in"=w495, "error in"=w494) -> ("task out"=w497:refnum<k21>, "error out"=w496:errorcluster)  [unwired: 12 in]
    }
  }
  n152 = Get Date/Time In Seconds() -> (seconds since 1Jan1904=w65:timestamp)
  n153 = case shown="False" w32 {
    tunnel: w31 -> [_ w501]
    tunnel: w30 -> [w498 w500]
    tunnel: [w498 w499] -> w22
    frame False {
    }
    frame True {
      n154 = VISA Close(VISA resource name=w501, error in (no error)=w500) -> (error out=w499:errorcluster)
    }
  }
  n155 = case shown="True" w44 {
    tunnel: w43 -> [_ w505]
    tunnel: w42 -> [w502 w504]
    tunnel: [w502 w503] -> w50
    frame False {
    }
    frame True {
      n156 = call <instrlib>:"Enable Output.vi"("error in (no error)"=w504, "Enable Output (T: Enable)"=FALSE, "VISA resource name"=w505) -> ("error out"=w506:errorcluster, "VISA resource name out"=w508:refnum<visa-resource-name>)  [unwired: 7 in]
      n157 = call <instrlib>:"Close.vi"("error in (no error)"=w506, "VISA resource name"=w508) -> ("error out"=w503:errorcluster)  [unwired: 9 in]
    }
  }
  n158 = case shown="True" w40 {
    tunnel: w38 -> [w509 w512]
    tunnel: [w509 w511] -> w51
    tunnel: w39 -> [_ w510]
    frame False {
    }
    frame True {
      n159 = call <instrlib>:"srsQcm200Close.vi"("error in"=w512, "Visa in"=w510) -> ("error out"=w511:errorcluster)  [unwired: 3 in]
    }
  }
  n160 = Format Date/Time String(seconds (now)=w65) -> (date/time string=→"Starting Date/Time":string)  [unwired: 2 in]
  n161 = case shown="True" w26 {
    tunnel: w25 -> [_ w516]
    tunnel: w24 -> [w513 w515]
    tunnel: [w513 w514] -> w23
    frame False {
    }
    frame True {
      n162 = VISA Close(VISA resource name=w516, error in (no error)=w515) -> (error out=w514:errorcluster)
    }
  }
  n163 = Unbundle(w2) -> ("error out"=w1:errorcluster)  [unwired: 2 out]
  n164 = Merge Errors(w23, w50, w51, w46, w22, w1) -> (w63:errorcluster)
  n165 = call <vilib>:"Simple Error Handler.vi"("error in (no error)"=w63) -> ("error out"=→"Program Errors":errorcluster)  [unwired: 4 in, 4 out]
  n166 = call <instrlib>:"OpenCreateReplace File.vi"("function (open:0)"=T3."create or replace") -> ("new file path"=w9:path)  [unwired: 7 in, 3 out]
  n167 = Build Array("date/time", "elapsed time (s)", "J-KEM temp (C)", "Keithley 2420 Resistance (Ohm)" ("element"), "QCM freq (Hz)", "QCM resistance (Ohm)", "O2 partial pressure (Torr)" ("element"), "O2 pump voltage (V)" ("element"), "Keithley 4200 4-point resistance (Ohm) " ("element"), "O2 concentration (%)" ("element"), "user comment" ("element")) -> (w12:string[])
  n168 = call-poly <vilib>:"Write To Spreadsheet File.vi"("1D data"=w12, "file path (dialog if empty)"=w9) -> ("new file path (Not A Path if cancelled)"=w13:path)  [unwired: 6 in]
  n169 = call-poly <vilib>:"Write To Spreadsheet File.vi"("append to file? (new file:F)"=TRUE, "2D data"=w62, "file path (dialog if empty)"=w13) -> ()  [unwired: 5 in, 1 out]
